vi "Move piece.vi"(8 "error in (no error)":errorcluster, 9 "Destination":T1={"File"=enum."a", "Rank"=enum."4"}, 10 "Source":T1={"File"=enum."a", "Rank"=enum."4"}, 11 "Position in":refnum<class "Position.lvclass">) -> (0 "error out":errorcluster, 1 "Captured piece":refnum<class "Piece.lvclass">, 2 "Capture?":bool, 3 "Position out":refnum<class "Position.lvclass">)   [LabVIEW 2016, in "Chesslib.lvlib" / "Position.lvclass"]
uses:
  Position.lvclass
  typedef/Square.ctl
  typedef/File.ctl
  typedef/Rank.ctl
  Pieces/Piece/Piece.lvclass
  Position.lvclass/Position.ctl
  Board/Board.lvclass
  Chesslib.lvlib
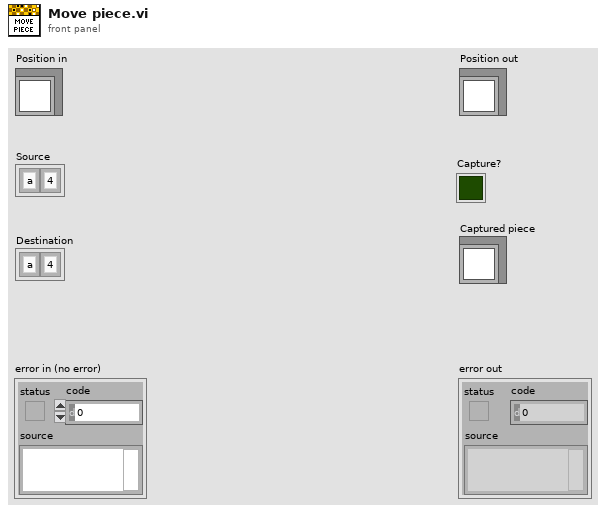
[diagram p1: front panel]
types:
  T1 = typedef "Chesslib.lvlib/Square.ctl" = cluster{"File":T2, "Rank":T3}
  T2 = typedef "Chesslib.lvlib/File.ctl" = enum8{"a", "b", "c", "d", "e", "f", "g", "h"}
  T3 = typedef "Chesslib.lvlib/Rank.ctl" = enum8{"1", "2", "3", "4", "5", "6", "7", "8"}
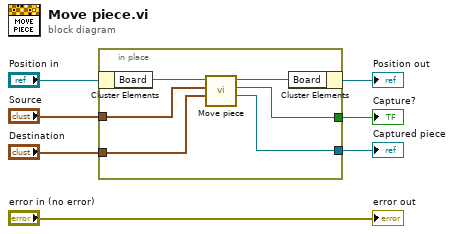
[diagram p0: block diagram]
diagram:
  n1 = in-place {
    in-place-border: "Source" -> [w11]
    in-place-border: "Destination" -> [w10]
    in-place-border: [w9] -> w2
    in-place-border: [w8] -> w1
    n2 = in-place-cluster #1("Position in") -> ("Board"=w13:refnum<class "Board.lvclass">)
    n3 = call "Move piece.vi"("Destination"=w10, "Source"=w11, "Board in"=w13) -> ("Removed piece"=w9:refnum<class "Piece.lvclass">, "Destination occupied?"=w8:bool, "Board out"=w12:refnum<class "Board.lvclass">)  [unwired: 6 in]
    n4 = in-place-cluster #1("Board"=w12) -> (→"Position out":refnum<class "Position.lvclass">)
  }
  "Capture?" <- w1
  "Captured piece" <- w2
  "error out" <- "error in (no error)"
